vi "Create User Event - Error.vi"(8 "error in (no error)":errorcluster) -> (0 "error out":errorcluster, 3 "UE Error":refnum<user-event>)   [LabVIEW 2017, in "User Events.lvlib"]
doc: "Create a Error user event that will be used to handle errors.."
uses:
  User Events.lvlib
  Error Handler/Controls/Error EventData.ctl
  Error Handler/Controls/Error Type.ctl
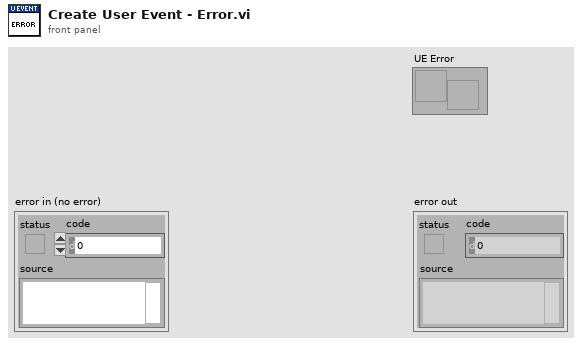
[diagram p1: front panel]
types:
  T1 = typedef "Error EventData.ctl" = cluster{"Error Type":T2, "error in (no error)":errorcluster}
  T2 = typedef "Error Type.ctl" = enum16{"Console Error", "Sensor Interface IO Error", "Process Step Error"}
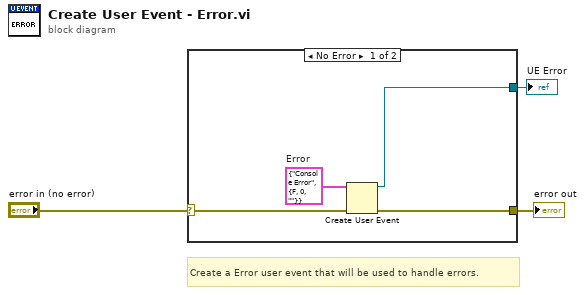
[diagram p0: block diagram]
diagram:
  # "Create a Error user event that will be used to handle errors."
  n1 = case shown="No Error" "error in (no error)" {
    selector: "error in (no error)" -> [w5 w8]
    tunnel: [w7 _] -> w1
    tunnel: [w6 w8] -> w3
    frame No Error {
      w4 = T1 {"Error Type"=enum."Console Error", "error in (no error)"={"status"=FALSE, "code"=0, "source"=""}}  # Error
      n2 = Create User Event(user event datatype=w4, error in=w5) -> (user event=w7:refnum<user-event>, error out=w6:errorcluster)
    }
    frame Error {
    }
  }
  "error out" <- w3
  "UE Error" <- w1
